vi "sv_Build Octave Info (1 Ch).vi"(0 "scaled signal [EU]":waveform(dbl), 5 "1/n octave settings":T2={"standard"=enum."ANSI S1.11", "bandwidth"=enum."1/3 octave"}, 7 "band number":cluster{"low band":i32, "high band":i32}, 11 "error in (no error)":errorcluster, 12 "channel index":i32) -> (3 "octave info":T3={"standard"=enum."ANSI S1.11", "bandwidth"=enum."1 octave", "low band"=0, "high band"=0, "weighting filter"=0, "dB reference"=0.0, "dB On"=FALSE, "unit label"="", "channel name"="", "description"="", "engineering units"=1, "custom label"="", "spectrum type"=enum."magnitude", "spectral density"=FALSE, "filters settled"=FALSE} {"engineering units" items=["custom..."=0, "V"=1, "A"=21, "C"=30, "pC"=31, "s"=32, "-"=29, "Pa"=2, "N"=20, "g"=3, "m/s^2"=4, "m/s"=5, "m"=6, "mm/s"=12, "mm"=13, "micron/s"=14, "micron"=15, "in/s^2"=7, "in/s"=8, "in"=9, "mil/s"=10, "mil"=11, "rad/s^2"=16, "rad/s"=17, "rad"=18, "deg/s^2"=26, "deg/s"=27, "deg"=28, "RPM"=22, "cycle/s^2"=23, "Hz"=24, "cycle"=25, "strain"=19]; "dB reference" format="%.2e"; "weighting filter" items=["Linear", "A-weighting", "B-weighting", "C-weighting", "ITU-R 468-4", "Dolby", "CCITT", "C-message", "Wb", "Wc", "Wd", "We", "Wf", "Wh", "Wj", "Wk", "Wm", "AES17 20 kHz lowpass", "AES17 40 kHz lowpass", "AES17 20 kHz highpass", "AES17 40 kHz highpass"]}, 4 "dup scaled signal [EU]":waveform(dbl), 6 "dup 1/n octave settings":T2={"standard"=enum."ANSI S1.11", "bandwidth"=enum."1/3 octave"}, 8 "dup band number":cluster{"low band":i32, "high band":i32}, 15 "error out":errorcluster)   [LabVIEW 2017, in "SoundVib_Octave_2014 standard.lvlib"]
uses:
  <vilib>/addons/Sound and Vibration/svt_Octave/SoundVib_Octave_2014 standard.lvlib
  <vilib>/addons/_NISVFA/_Shared subVIs/Controls/svc_Octave Standard.ctl
  <vilib>/addons/_NISVFA/_Shared subVIs/Controls/svc_Octave Info.ctl
  <vilib>/addons/_NISVFA/_Shared subVIs/Controls/svc_Weighting Filter Text Ring.ctl
  <vilib>/addons/_NISVFA/_Shared subVIs/Controls/svc_Engineering Units Text Ring.ctl
  <vilib>/addons/_NISVFA/_Shared subVIs/Common/svc_Engineering Units to Unit Label.vi
  <vilib>/addons/_NISVFA/_Shared subVIs/Common/svc_Unit Label to Engineering Units.vi
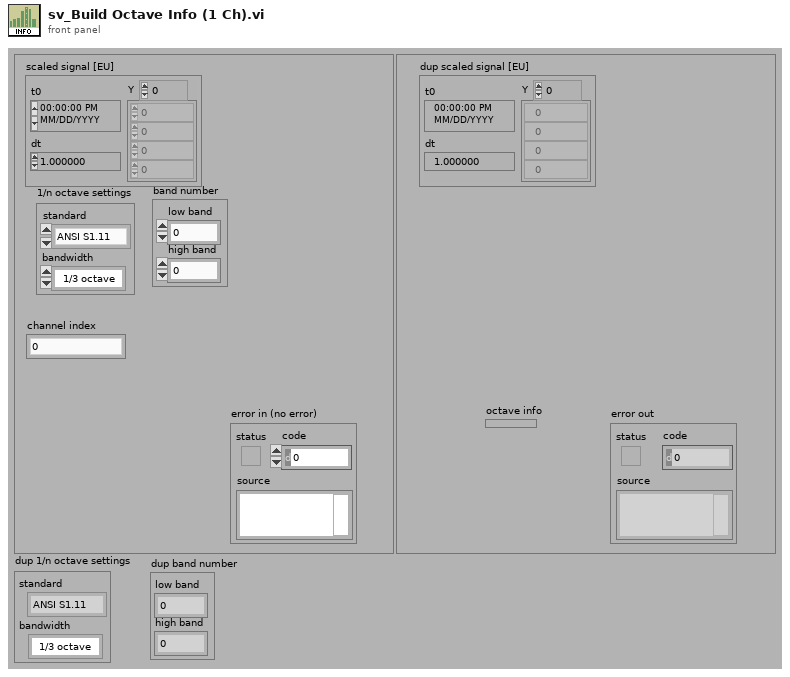
[diagram p1: front panel]
types:
  T1 = typedef "svc_Octave Standard.ctl" = enum16{"ANSI S1.11", "IEC 61260"}
  T2 = cluster{"standard":T1, "bandwidth":enum16{"1 octave", "1/3 octave", "1/6 octave", "1/12 octave", "1/24 octave"}}
  T3 = typedef "svc_Octave Info.ctl" = cluster{"standard":T1, "bandwidth":enum16{"1 octave", "1/3 octave", "1/6 octave", "1/12 octave", "1/24 octave"}, "low band":i32, "high band":i32, "weighting filter":T4, "dB reference":dbl, "dB On":bool, "unit label":string, "channel name":string, "description":string, "engineering units":T5, "custom label":string, "spectrum type":enum16{"power", "magnitude"}, "spectral density":bool, "filters settled":bool}
  T4 = typedef "svc_Weighting Filter Text Ring.ctl" = u16
  T5 = typedef "svc_Engineering Units Text Ring.ctl" = u16
  T6 = typedef "svc_Channel Info.ctl" = cluster{"sensor sensitivity":dbl, "engineering units":T5, "dB reference":dbl, "custom label":string, "weighting filter":T4, "pregain":dbl}
  T7 = enum16{"1 octave", "1/3 octave", "1/6 octave", "1/12 octave", "1/24 octave"}
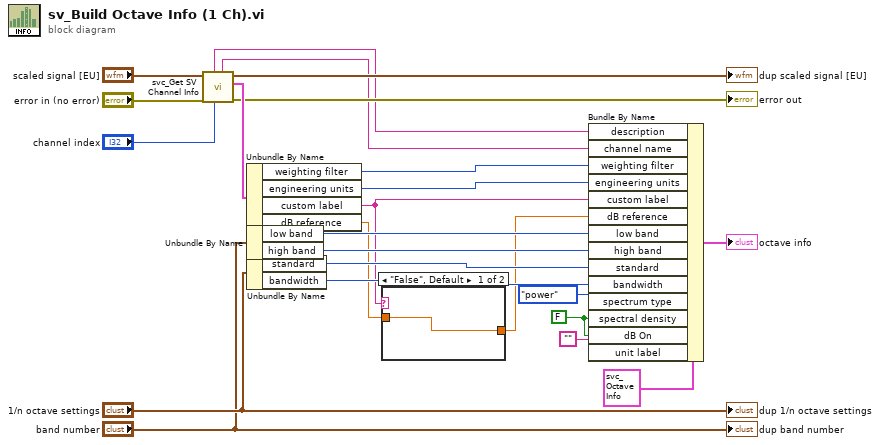
[diagram p0: block diagram]
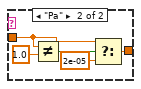
[diagram p2: hidden frame]
diagram:
  w10 = FALSE ("dB On")
  n1 = call <vilib>:"svc_Get SV Channel Info.vi"("channel index"="channel index", "error in (no error)"="error in (no error)", "scaled signal [EU]"="scaled signal [EU]") -> ("error out"=→"error out":errorcluster, "channel info"=w19:T6, "dup scaled signal [EU]"=→"dup scaled signal [EU]":waveform(dbl), "channel name"=w14:string, "channel description"=w13:string)  [unwired: 3 in, 1 out]
  n2 = Unbundle By Name(w19) -> ("weighting filter"=w7:T4, "engineering units"=w11:T5, "custom label"=w5:string, "dB reference"=w4:dbl)
  n3 = Unbundle By Name("band number") -> ("low band"=w6:i32, "high band"=w15:i32)
  n4 = Unbundle By Name("1/n octave settings") -> ("standard"=w17:T1, "bandwidth"=w16:T7)
  n5 = case shown="\"False\", Default" w5 {
    tunnel: w4 -> [w25 w27]
    tunnel: [w25 w26] -> w3
    frame "False", Default {
    }
    frame "Pa" {
      n6 = Not Equal?(x=w27, y=1.0) -> (x != y?=w29:bool)
      n7 = Select(t=w27, s=w29, f=2e-05 ("y")) -> (s? t:f=w26:dbl)
    }
  }
  n8 = Bundle By Name(cluster=T3 {"standard"=enum."ANSI S1.11", "bandwidth"=enum."1 octave", "low band"=0, "high band"=0, "weighting filter"=0, "dB reference"=0.0, "dB On"=FALSE, "unit label"="", "channel name"="", "description"="", "engineering units"=1, "custom label"="", "spectrum type"=enum."magnitude", "spectral density"=FALSE, "filters settled"=FALSE} ("octave info"), "description"=w13, "channel name"=w14, "weighting filter"=w7, "engineering units"=w11, "custom label"=w5, "dB reference"=w3, "low band"=w6, "high band"=w15, "standard"=w17, "bandwidth"=w16, "spectrum type"=enum16{"power", "magnitude"}."power", "spectral density"=w10, "dB On"=w10, "unit label"="") -> (→"octave info":T3)
  "dup 1/n octave settings" <- "1/n octave settings"
  "dup band number" <- "band number"
